vi "Query Each Found Address.vi"(8 "error in (no error) 2":errorcluster, 11 "Address":string) -> (0 "error out (no error)":errorcluster, 2 "read buffer":string)   [LabVIEW 2014, in "SetUp VIs.lvlib"]
uses:
  SetUp VIs.lvlib
  <instrlib>/Fluke 2625A/Fluke 2625A.lvlib
panel:
  out "STOP COUNTER":i32
  out "VISA resource name out 2":refnum<visa-resource-name>
  in  "manual?":bool
  out "Interface Information:Interface Type":u16
  in  "VISA resource name out":refnum<visa-resource-name>
  out "return count":u32
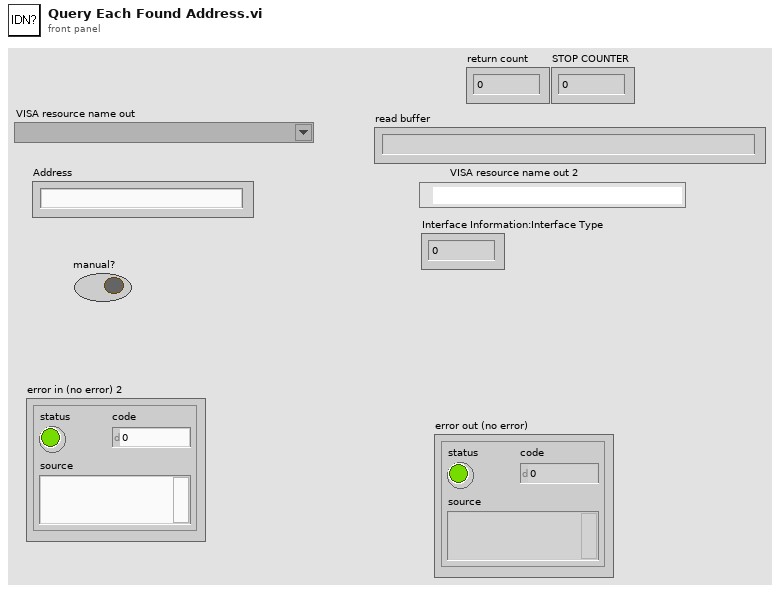
[diagram p1: front panel]
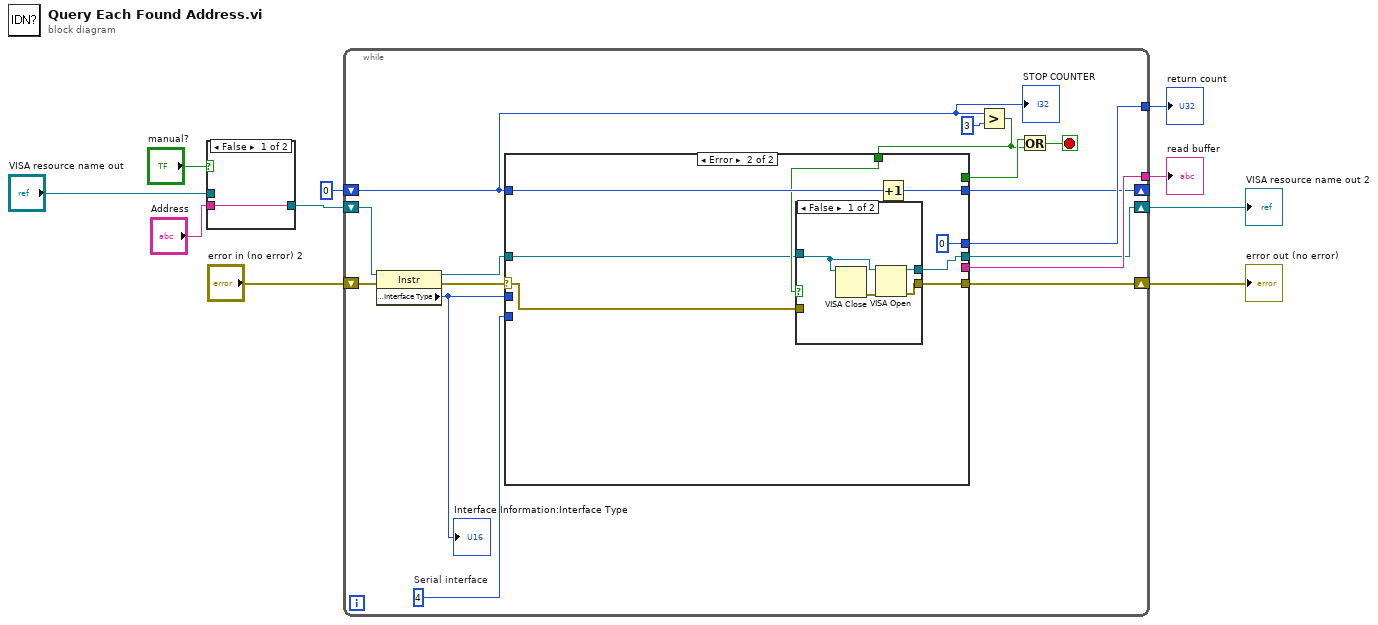
[diagram p0: block diagram]
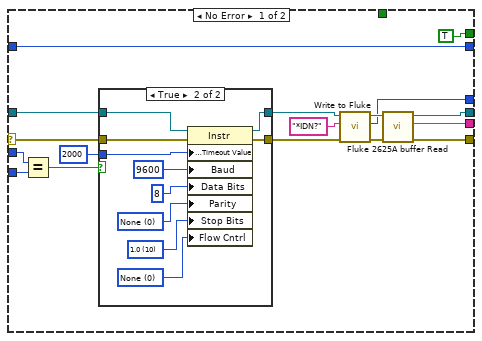
[diagram p2: hidden frame]
diagram:
  n1 = case shown="False" "manual?" {
    tunnel: [w11 w12] -> w1
    tunnel: "VISA resource name out" -> [_ w12]
    tunnel: "Address" -> [w11 _]
    frame False {
    }
    frame True {
    }
  }
  n2 = while {
    tunnel: [w28] -> w10
    tunnel: [w23] -> w8
    shift-right: [w22] -> w4
    shift-left: w1 -> [w21]
    shift-right: [w27] -> w9
    shift-left: "error in (no error) 2" -> [w20]
    shift-right: [w16] -> _
    shift-left: 0 -> [w15]
    stop <- w18 stop-if-true
    w24 = u16 4  # Serial interface
    n3 = property class="Instr"(reference=w21, error in=w20) -> (reference out=w26:refnum<visa-resource-name>, error out=w19:errorcluster, "Interface Information:Interface Type"=w25:u16)
    "Interface Information:Interface Type" <- w25
    n4 = Greater?(x=w15, y=3) -> (0:w13:bool)
    n5 = case shown="Error" w19 {
      selector: w19 -> [w31 w60]
      tunnel: [w43 u32 0 ("return count")] -> w28
      tunnel: [w42 w62] -> w27
      tunnel: w26 -> [w41 w58]
      tunnel: w25 -> [w39 _]
      tunnel: w24 -> [w38 _]
      tunnel: [w34 _] -> w23
      tunnel: [w32 w59] -> w22
      tunnel: [TRUE _] -> w17
      tunnel: w15 -> [w29 w64]
      tunnel: [w29 w63] -> w16
      tunnel: w13 -> [_ w61]
      frame No Error {
        n6 = Equal?(x=w39, y=w38) -> (x = y?=w40:bool)
        n7 = case shown="True" w40 {
          tunnel: [w46 w55] -> w37
          tunnel: [w47 w54] -> w36
          tunnel: w41 -> [w46 w57]
          tunnel: w31 -> [w47 w56]
          tunnel: u32 2000 ("Tmo Value") -> [_ w53]
          frame False {
          }
          frame True {
            w48 = u16 0 items=["None", "XON/XOFF", "RTS/CTS", "XON/XOFF & RTS/CTS", "DTR/DSR", "XON/XOFF & DTR/DSR"] ("Serial Settings:Flow Control")
            w49 = u16 10 items=["1.0"=10, "1.5"=15, "2.0"=20] ("Serial Settings:Stop Bits")
            w50 = u16 0 items=["None", "Odd", "Even", "Mark", "Space"] ("Serial Settings:Parity")
            n8 = property class="Instr"(reference=w57, error in=w56, "General Settings:Timeout Value"=w53, "Baud"=u32 9600 ("Serial Settings:Baud Rate"), "Data Bits"=u16 8 ("Serial Settings:Data Bits"), "Parity"=w50, "Stop Bits"=w49, "Flow Cntrl"=w48) -> (reference out=w55:refnum<visa-resource-name>, error out=w54:errorcluster)
          }
        }
        n9 = call <instrlib>:"Write to Fluke.vi"("error in (no error)"=w36, "write buffer"="*IDN?", "VISA resource name"=w37) -> ("error out"=w45:errorcluster, "return count"=w43:u32, "VISA resource name 2"=w44:refnum<visa-resource-name>)  [unwired: 6 in]
        n10 = call <instrlib>:"Fluke 2625A buffer Read.vi"("error out"=w45, "VISA resource name out"=w44) -> ("error out 2"=w42:errorcluster, "read buffer"=w34:string, "VISA resource name out 2"=w32:refnum<visa-resource-name>)  [unwired: 7 in]
      }
      frame Error {
        n11 = case shown="False" w61 {
          tunnel: w58 -> [w67 w70]
          tunnel: [w68 w71] -> w62
          tunnel: w60 -> [_ w71]
          tunnel: [w66 w70] -> w59
          frame False {
            n12 = VISA Close(VISA resource name=w67) -> (error out=w69:errorcluster)  [unwired: 1 in]
            n13 = VISA Open(error in (no error)=w69, VISA resource name=w67) -> (VISA resource name=w66:refnum<visa-resource-name>, error out=w68:errorcluster)  [unwired: 3 in]
          }
          frame True {
          }
        }
        n14 = Increment(x=w64) -> (x+1=w63:i32)
      }
    }
    n15 = Or(x=w17, y=w13) -> (x .or. y?=w18:bool)
    "STOP COUNTER" <- w15
  }
  "error out (no error)" <- w9
  "read buffer" <- w8
  "return count" <- w10
  "VISA resource name out 2" <- w4
